vi "MVE Export.vi"(11 "Full Path":string) -> (0 "error out":errorcluster, 3 "cancelled":bool)   [LabVIEW 2016]
uses:
  <resource>/dialog/variable/SCT Variable.ctl
  <vilib>/variable/Type Descriptor.ctl
  <vilib>/variable/Attribs.ctl
  <vilib>/variable/NI_Variable.lvlib
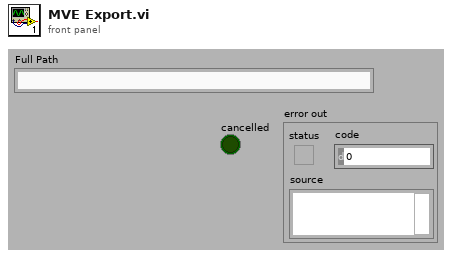
[diagram p1: front panel]
types:
  T1 = typedef "SCT Variable.ctl" = cluster{"Name":string, "TypeDesc":T2, "Type":string, "typedefs":string, "Attribs":T3, "FeaturePacks":string[], "Source":string}
  T2 = typedef "NI_Variable.lvlib/Type Descriptor.ctl" = cluster{"Variant":variant}
  T3 = typedef "NI_Variable.lvlib/Attribs.ctl" = cluster{"Attrib":string, "Value":string}[]
  T4 = typedef "NI_Variable.lvlib/variable.ctl" = cluster{"Name":string, "TypeDesc":T2, "Type":string, "Typedefs":string, "Attribs":T3, "FeaturePacks":string[]}
  T5 = typedef "SCT Default Types.ctl" = cluster{"names":string[], "TDs":T2[]}
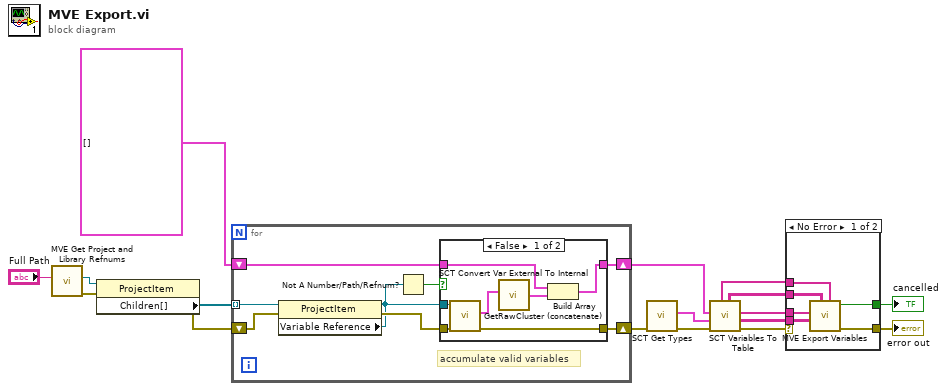
[diagram p0: block diagram]
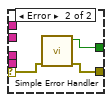
[diagram p2: hidden frame]
diagram:
  n1 = call <resource>:"MVE Get Project and Library Refnums.vi"("Full Path"="Full Path") -> ("error out"=w15:errorcluster, "ProjectItem Refnum"=w3:refnum<vi>)  [unwired: 8 in, 1 out]
  n2 = property class="ProjectItem"(reference=w3, error in=w15) -> (error out=w14:errorcluster, "Children[]"=w16:refnum<vi>[])  [unwired: 1 out]
  n3 = for {
    tunnel: w16 -> [w24] mode=indexing
    shift-right: [w25] -> w12
    shift-left: w14 -> [w22]
    shift-right: [w20] -> w10
    shift-left: T1[] [] -> [w19]
    # "accumulate valid variables"
    n4 = property class="ProjectItem"(reference=w24, error in=w22) -> (error out=w23:errorcluster, "Variable Reference"=w21:refnum<vi>)  [unwired: 1 out]
    n5 = Not A Number/Path/Refnum?(number/path/refnum=w21) -> (NaN/Path/Refnum?=w18:bool)
    n6 = case shown="False" w18 {
      tunnel: [w32 w33] -> w25
      tunnel: w23 -> [w31 w33]
      tunnel: w21 -> [w28 _]
      tunnel: [w27 w34] -> w20
      tunnel: w19 -> [w26 w34]
      frame False {
        n7 = call <vilib>:"GetRawCluster.vi"("error in (no error)"=w31, "Variable Reference in"=w28) -> ("error out"=w32:errorcluster, "Variable"=w30:T4)  [unwired: 7 in, 1 out]
        n8 = call <resource>:"SCT Convert Var External To Internal.vi"("External Var"=w30) -> ("Internal Var"=w29:T1)  [unwired: 5 in]
        n9 = Build Array (concatenate)(w26, w29) -> (w27:T1[])
      }
      frame True {
      }
    }
  }
  n10 = call <resource>:"SCT Get Types.vi"("error in"=w12) -> ("error out"=w11:errorcluster, "default types"=w13:T5)  [unwired: 8 in, 1 out]
  n11 = call <resource>:"SCT Variables To Table.vi"("error in (no error)"=w11, "default types"=w13, "variables"=w10) -> ("error out"=w9:errorcluster, "DisplayedTable"=w8:string[][], "DisplayedHeader"=w7:string[], "Filtered Table"=w6:string[][], "Filtered Header"=w5:string[])  [unwired: 4 in]
  n12 = case shown="No Error" w9 {
    selector: w9 -> [_ w43]
    tunnel: w8 -> [w40 _]
    tunnel: w7 -> [w39 _]
    tunnel: w6 -> [w38 _]
    tunnel: w5 -> [w37 _]
    tunnel: [w36 w42] -> w2
    tunnel: [w35 w41] -> w1
    frame No Error {
      n13 = call <resource>:"MVE Export Variables.vi"("FilterHeader"=w37, "FilterContent"=w38, "Item Names"=w40, "Prop Names"=w39) -> ("error out"=w36:errorcluster, "cancelled"=w35:bool)  [unwired: 6 in]
    }
    frame Error {
      n14 = call <vilib>:"Simple Error Handler.vi"("error in (no error)"=w43) -> ("error?"=w41:bool, "error out"=w42:errorcluster)  [unwired: 4 in, 3 out]
    }
  }
  "error out" <- w2
  "cancelled" <- w1
